vi "Current State.vi"(8 "error in (no error)":errorcluster, 10 "Motors with Encoder State":T1={"Forward Switch"=FALSE, "Reverse Switch"=FALSE, "Measured RPM"=0.0, "Distance (in)"=0.0, "Setpoint RPM"=0.0, "Encoder Count"=0, "Home Count"=0, "Config"={"Counts  Per Revolution"=0, "Invert Encoder Direction"=FALSE, "Diameter of Revolution"=0.0, "Max RPM"=0.0, "Encoder Control"=TRUE}}, 11 "Motors with Encoders in":refnum<class "Motors with Encoders.lvclass">) -> (0 "error out":errorcluster, 3 "Motors with Encoders out":refnum<class "Motors with Encoders.lvclass">)   [LabVIEW 2014, in "Motors with Encoders.lvlib" / "Motors with Encoders.lvclass"]
uses:
  Motors with Encoders.lvclass
  Motors with Encoders State.ctl
  Motors with Encoders Config.ctl
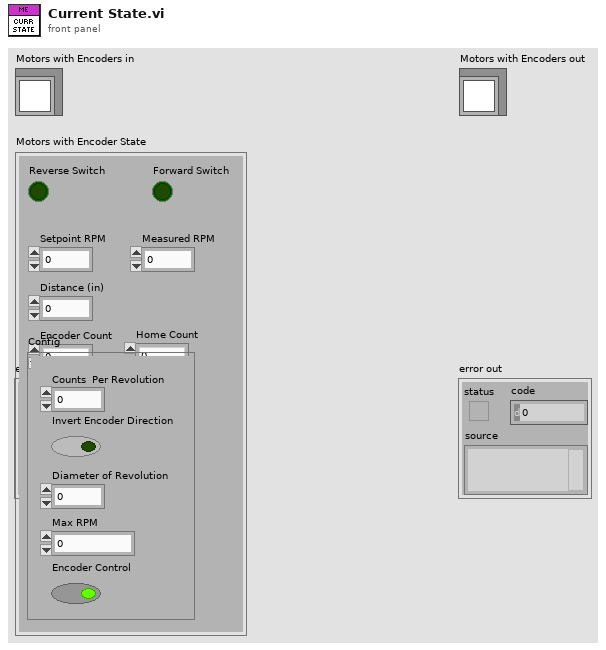
[diagram p1: front panel]
types:
  T1 = typedef "Motors with Encoders.lvlib/Motors with Encoders.lvclass/Motors with Encoders State.ctl" = cluster{"Forward Switch":bool, "Reverse Switch":bool, "Measured RPM":dbl, "Distance (in)":dbl, "Setpoint RPM":dbl, "Encoder Count":i64, "Home Count":i64, "Config":T2}
  T2 = typedef "Motors with Encoders.lvlib/Motors with Encoders.lvclass/Motors with Encoders Config.ctl" = cluster{"Counts  Per Revolution":u32, "Invert Encoder Direction":bool, "Diameter of Revolution":dbl, "Max RPM":dbl, "Encoder Control":bool}
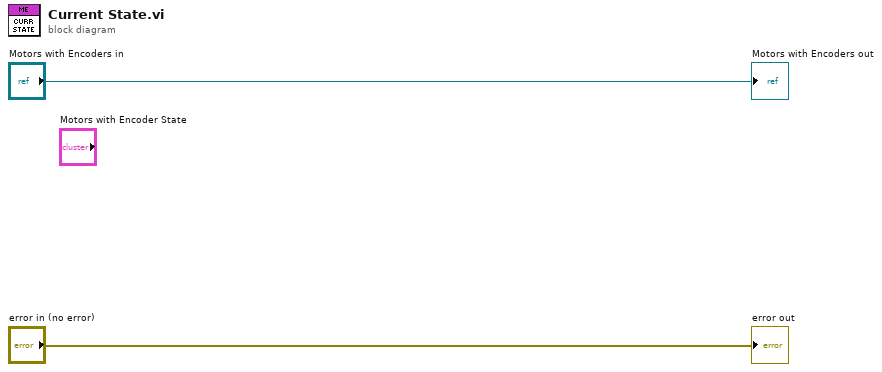
[diagram p0: block diagram]
diagram:
  "error out" <- "error in (no error)"
  "Motors with Encoders out" <- "Motors with Encoders in"
